vi "DHE_DRV_get_info.vi"(0 "fd":i32, 5 "get pci info?":bool, 11 "error in (no error)":errorcluster) -> (4 "fd":i32, 6 "Info":u16[](array[numeric]), 8 "error_code":i32, 15 "error out":errorcluster)   [LabVIEW 2016]
doc: "This VI closes the I/O interface with the instrument."
uses:
  c/lib/libarcDHE.so
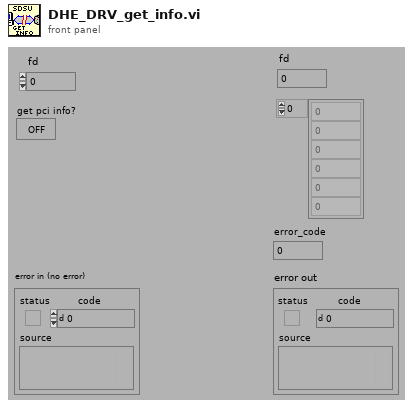
[diagram p1: front panel]
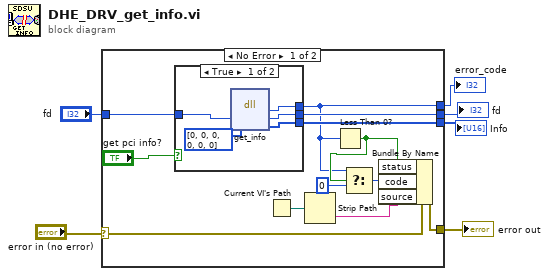
[diagram p0: block diagram]
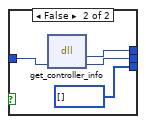
[diagram p2: hidden frame]
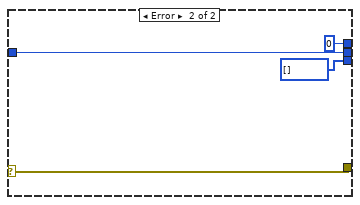
[diagram p3: hidden frame]
diagram:
  n1 = case shown="No Error" "error in (no error)" {
    selector: "error in (no error)" -> [w12 w28]
    tunnel: "fd" -> [w18 w31]
    tunnel: [w9 0] -> w5
    tunnel: [w15 w28] -> w4
    tunnel: [w14 w31] -> w3
    tunnel: [w13 u16[] [] ("info")] -> w2
    frame No Error {
      n2 = case shown="True" "get pci info?" {
        tunnel: w18 -> [w23 w27]
        tunnel: [w22 w26] -> w9
        tunnel: [w21 w25] -> w14
        tunnel: [w20 u16[] [] ("info")] -> w13
        frame True {
          n3 = dll-call lib="home/simager/panview/PAN/Modules/SDSU/private/c/lib/libarcDHE.so" fn="get_info"("fd"=w23, "info"=u16[] [0, 0, 0, 0, 0, 0] ("Array Constant")) -> (w22:i32, "fd"=w21:i32, "info"=w20:u16[])  [unwired: 3 in, 2 out]
        }
        frame False {
          n4 = dll-call lib="home/simager/panview/PAN/Modules/SDSU/private/c/lib/libarcDHE.so" fn="get_controller_info"("fd"=w27) -> (w26:i32, "fd"=w25:i32)  [unwired: 3 in, 2 out]
        }
      }
      n5 = Current VI's Path() -> (path=w17:path)
      n6 = Strip Path(path=w17) -> (name=w16:string)  [unwired: 1 out]
      n7 = Less Than 0?(x=w9) -> (x < 0?=w10:bool)
      n8 = Select(t=w9, s=w10, f=0) -> (s? t:f=w7:i32)
      n9 = Bundle By Name(cluster=w12, "status"=w10, "code"=w7, "source"=w16) -> (w15:errorcluster)
    }
    frame Error {
    }
  }
  "error out" <- w4
  "error_code" <- w5
  "fd" <- w3
  "Info" <- w2
